vi "RunProgramOnBrick_Modified.vi"(8 "error in (no error)":errorcluster, 10 "Program Name":string, 11 "VIA in":refnum<class "VIA.lvclass">=refnum) -> (0 "error out":errorcluster, 3 "VIA out":refnum<class "VIA.lvclass">)   [LabVIEW 2014]
uses:
  <vilib>/NXT/LegoClasses/VIA/VIA.lvclass
panel:
  out "error out 2":errorcluster
  out "standard error":string
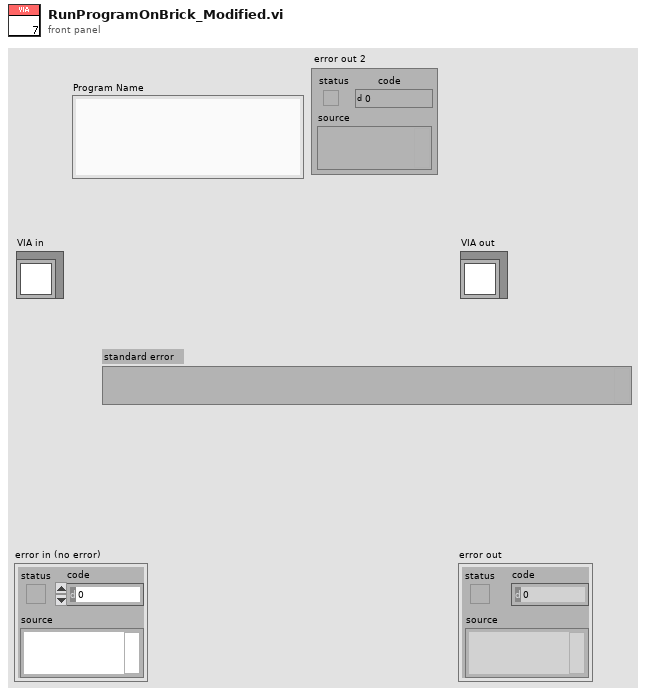
[diagram p1: front panel]
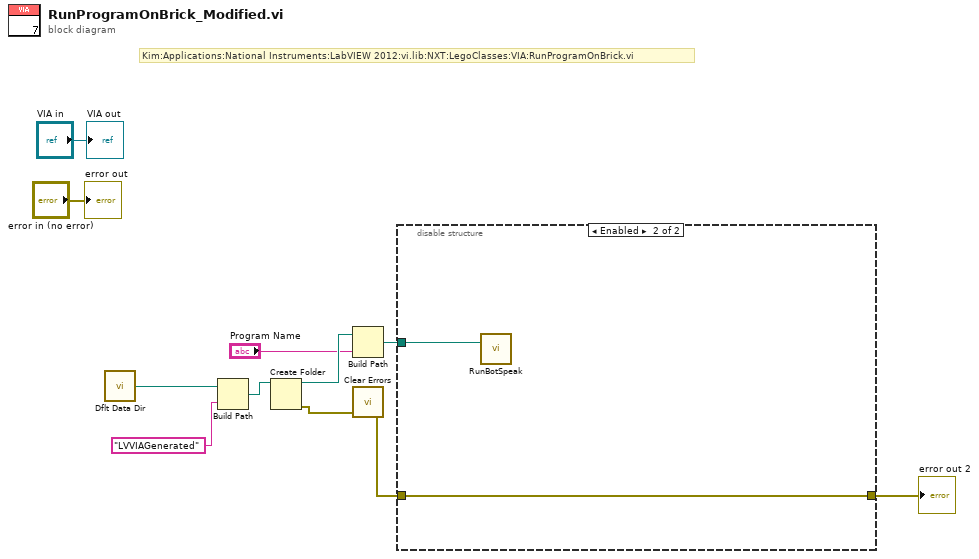
[diagram p0: block diagram]
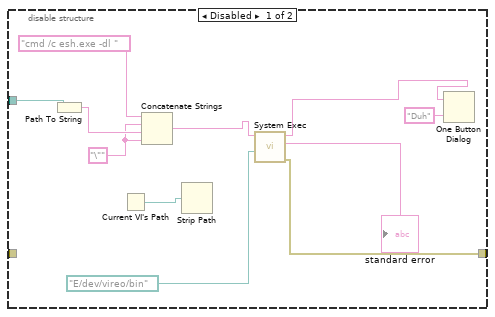
[diagram p2: hidden frame]
diagram:
  # "Kim:Applications:National Instruments:LabVIEW 2012:vi.lib:NXT:LegoClasses:VIA:RunProgramOnBrick.vi"
  n1 = call <vilib>:"Dflt Data Dir.vi"() -> ("App:Default Data Directory"=w11:path)
  n2 = Build Path(base path=w11, name or relative path="LVVIAGenerated" ("file (use dialog)")) -> (appended path=w10:path)
  n3 = Create Folder(path (use dialog)=w10) -> (created path=w3:path, error out=w8:errorcluster)  [unwired: 2 in, 1 out]
  n4 = Build Path(base path=w3, name or relative path="Program Name") -> (appended path=w1:path)
  n5 = call <vilib>:"Clear Errors.vi"("error in (no error)"=w8) -> ("error out"=w4:errorcluster)  [unwired: 5 in, 1 out]
  n6 = disable-structure shown="Enabled" {
    disable-tunnel: [w13 w24] -> w5
    disable-tunnel: w4 -> [_ w24]
    disable-tunnel: w1 -> [w12 w23]
    frame Disabled {
      w20 = "\"" ("string")
      n7 = Path To String(path=w12) -> (string=w21:string)
      n8 = Current VI's Path() -> (path=w22:path)
      n9 = Concatenate Strings("cmd /c esh.exe -dl " ("string"), w20, w21, w20) -> (w17:string)
      n10 = Strip Path(path=w22) -> ()  [unwired: 2 out]
      n11 = call <vilib>:"System Exec.vi"("working directory"=path "E:/dev/vireo/bin" ("stripped path"), "command line"=w17) -> ("error out"=w13:errorcluster, "standard error"=→"standard error":string, "standard output"=w16:string)  [unwired: 6 in, 1 out]
      n12 = One Button Dialog(message=w16, button name ("OK")="Duh") -> ()  [unwired: 1 out]
    }
    frame Enabled {
      n13 = call <vilib>:"RunBotSpeak.vi"("VIA"=w23) -> ()  [unwired: 3 in]
    }
  }
  "error out 2" <- w5
  "error out" <- "error in (no error)"
  "VIA out" <- "VIA in"
